vi "EventLog.CreateError.vi"   [LabVIEW 2016]
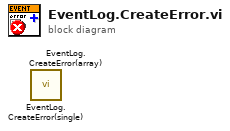
[diagram p0: block diagram]
diagram:
  n1 = call "EventLog.CreateError(single).vi"() -> ()  [unwired: 11 in, 1 out]
  n2 = call "EventLog.CreateError(array).vi"() -> ()  [unwired: 10 in, 2 out]
